vi "ValueChangeTest.vi"() -> ()   [LabVIEW 2016]
uses:
  <vilib>/addons/_JKI Toolkits/Caraya/classes/Assert/Assert Equal Value and Type_Variant.vi
  <vilib>/addons/_JKI Toolkits/Caraya/classes/Assert/Assert.lvclass
  <vilib>/addons/_JKI Toolkits/Caraya/classes/Test/Test.lvclass
panel:
  out "error out":errorcluster
  in  "error in":errorcluster
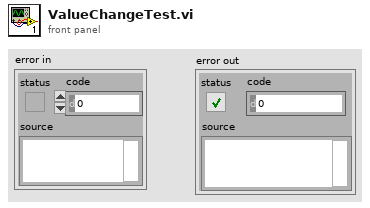
[diagram p1: front panel]
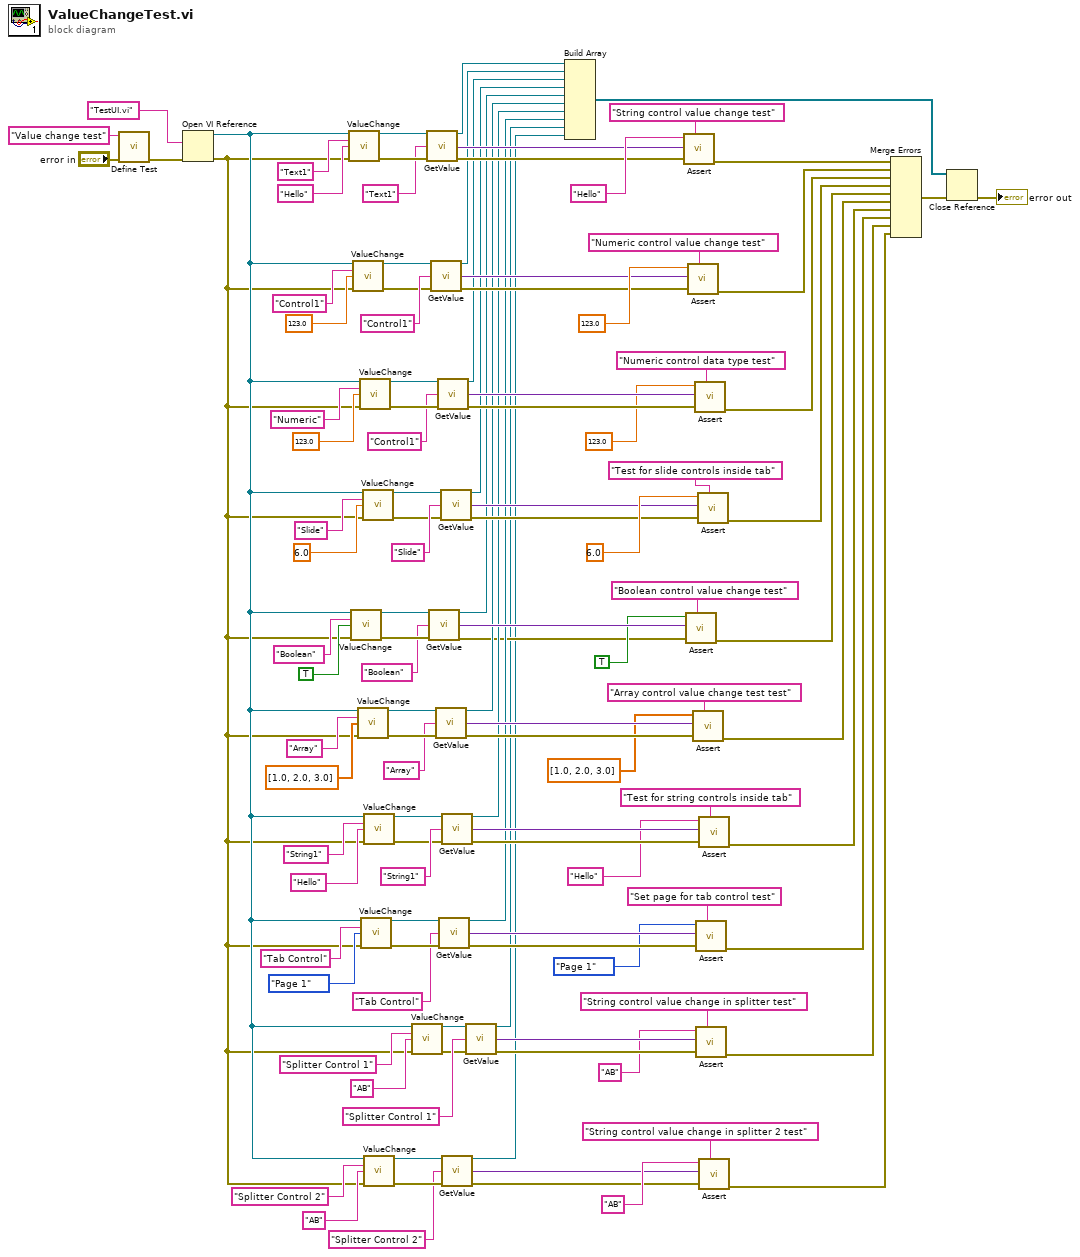
[diagram p0: block diagram]
diagram:
  n1 = call <vilib>:"Define Test.vi"("error in (no error)"="error in", "Label (VI Title)"="Value change test") -> ("error out"=w111:errorcluster)  [unwired: 9 in]
  n2 = Open VI Reference(vi path="TestUI.vi", error in (no error)=w111) -> (vi reference=w4:refnum<vi>, error out=w3:errorcluster)  [unwired: 4 in]
  n3 = call "ValueChange.vi"("VI Reference"=w4, "Control Name"="Text1", "Value"="Hello" ("Control Name"), "error in"=w3) -> ("reference out"=w109:refnum<vi>, "error out"=w118:errorcluster)  [unwired: 10 in]
  n4 = call "ValueChange.vi"("VI Reference"=w4, "Control Name"="Boolean", "Value"=TRUE, "error in"=w3) -> ("reference out"=w73:refnum<vi>, "error out"=w72:errorcluster)  [unwired: 10 in]
  n5 = call "ValueChange.vi"("VI Reference"=w4, "Control Name"="Control1", "Value"=123.0 ("Control Name"), "error in"=w3) -> ("reference out"=w102:refnum<vi>, "error out"=w103:errorcluster)  [unwired: 10 in]
  n6 = call "ValueChange.vi"("VI Reference"=w4, "Control Name"="Array", "Value"=dbl[] [1.0, 2.0, 3.0], "error in"=w3) -> ("reference out"=w63:refnum<vi>, "error out"=w62:errorcluster)  [unwired: 10 in]
  n7 = call "ValueChange.vi"("VI Reference"=w4, "Control Name"="Numeric", "Value"=123.0 ("Control Name"), "error in"=w3) -> ("reference out"=w93:refnum<vi>, "error out"=w92:errorcluster)  [unwired: 10 in]
  n8 = call "ValueChange.vi"("VI Reference"=w4, "Control Name"="Tab Control", "Value"=enum32{"Page 1", "Page 2", "Page 3"}."Page 1" ("Tab Control"), "error in"=w3) -> ("reference out"=w33:refnum<vi>, "error out"=w32:errorcluster)  [unwired: 10 in]
  n9 = call "ValueChange.vi"("VI Reference"=w4, "Control Name"="Slide", "Value"=6.0 ("Control Name"), "error in"=w3) -> ("reference out"=w80:refnum<vi>, "error out"=w81:errorcluster)  [unwired: 10 in]
  n10 = call "ValueChange.vi"("VI Reference"=w4, "Control Name"="String1", "Value"="Hello" ("Control Name"), "error in"=w3) -> ("reference out"=w53:refnum<vi>, "error out"=w54:errorcluster)  [unwired: 10 in]
  n11 = call "ValueChange.vi"("VI Reference"=w4, "Control Name"="Splitter Control 2", "Value"="AB", "error in"=w3) -> ("reference out"=w9:refnum<vi>, "error out"=w8:errorcluster)  [unwired: 10 in]
  n12 = call "ValueChange.vi"("VI Reference"=w4, "Control Name"="Splitter Control 1", "Value"="AB", "error in"=w3) -> ("reference out"=w21:refnum<vi>, "error out"=w22:errorcluster)  [unwired: 10 in]
  n13 = call "GetValue.vi"("VI Reference"=w109, "Control Name"="Text1", "error in"=w118) -> ("VI Reference out"=w44:refnum<vi>, "Control Value"=w100:variant, "error out"=w101:errorcluster)  [unwired: 10 in]
  n14 = call "GetValue.vi"("VI Reference"=w73, "Control Name"="Boolean", "error in"=w72) -> ("VI Reference out"=w39:refnum<vi>, "Control Value"=w74:variant, "error out"=w28:errorcluster)  [unwired: 10 in]
  n15 = call "GetValue.vi"("VI Reference"=w102, "Control Name"="Control1", "error in"=w103) -> ("VI Reference out"=w42:refnum<vi>, "Control Value"=w98:variant, "error out"=w99:errorcluster)  [unwired: 10 in]
  n16 = call "GetValue.vi"("VI Reference"=w63, "Control Name"="Array", "error in"=w62) -> ("VI Reference out"=w38:refnum<vi>, "Control Value"=w65:variant, "error out"=w64:errorcluster)  [unwired: 10 in]
  n17 = call "GetValue.vi"("VI Reference"=w93, "Control Name"="Control1", "error in"=w92) -> ("VI Reference out"=w41:refnum<vi>, "Control Value"=w95:variant, "error out"=w94:errorcluster)  [unwired: 10 in]
  n18 = call "GetValue.vi"("VI Reference"=w33, "Control Name"="Tab Control", "error in"=w32) -> ("VI Reference out"=w29:refnum<vi>, "Control Value"=w35:variant, "error out"=w34:errorcluster)  [unwired: 10 in]
  n19 = call "GetValue.vi"("VI Reference"=w80, "Control Name"="Slide", "error in"=w81) -> ("VI Reference out"=w40:refnum<vi>, "Control Value"=w78:variant, "error out"=w79:errorcluster)  [unwired: 10 in]
  n20 = call "GetValue.vi"("VI Reference"=w53, "Control Name"="String1", "error in"=w54) -> ("VI Reference out"=w37:refnum<vi>, "Control Value"=w51:variant, "error out"=w52:errorcluster)  [unwired: 10 in]
  n21 = call "GetValue.vi"("VI Reference"=w9, "Control Name"="Splitter Control 2", "error in"=w8) -> ("VI Reference out"=w2:refnum<vi>, "Control Value"=w11:variant, "error out"=w10:errorcluster)  [unwired: 10 in]
  n22 = call "GetValue.vi"("VI Reference"=w21, "Control Name"="Splitter Control 1", "error in"=w22) -> ("VI Reference out"=w15:refnum<vi>, "Control Value"=w19:variant, "error out"=w20:errorcluster)  [unwired: 10 in]
  n23 = Build Array(w44, w42, w41, w40, w39, w38, w37, w29, w15, w2) -> (w43:refnum<vi>[])
  n24 = call-poly <vilib>:"Assert.vi"("Label"="String control value change test", "error in (no error)"=w101, "Y"=w100, "X"="Hello" ("Control Name")) -> ("error out"=w97:errorcluster)  [unwired: 7 in]
  n25 = call-poly <vilib>:"Assert.vi"("Label"="Boolean control value change test", "error in (no error)"=w28, "Y"=w74, "X"=TRUE) -> ("error out"=w68:errorcluster)  [unwired: 7 in]
  n26 = call-poly <vilib>:"Assert.vi"("Label"="Numeric control value change test", "error in (no error)"=w99, "Y"=w98, "X"=123.0 ("Control Name")) -> ("error out"=w96:errorcluster)  [unwired: 7 in]
  n27 = call-poly <vilib>:"Assert.vi"("Label"="Array control value change test test", "error in (no error)"=w64, "Y"=w65, "X"=dbl[] [1.0, 2.0, 3.0]) -> ("error out"=w57:errorcluster)  [unwired: 7 in]
  n28 = call-poly <vilib>:"Assert.vi"("Label"="Numeric control data type test", "error in (no error)"=w94, "Y"=w95, "X"=123.0 ("Control Name")) -> ("error out"=w86:errorcluster)  [unwired: 7 in]
  n29 = call-poly <vilib>:"Assert.vi"("Label"="Set page for tab control test", "error in (no error)"=w34, "Y"=w35, "X"=enum32{"Page 1", "Page 2", "Page 3"}."Page 1" ("Tab Control")) -> ("error out"=w27:errorcluster)  [unwired: 7 in]
  n30 = call-poly <vilib>:"Assert.vi"("Label"="String control value change in splitter test", "error in (no error)"=w20, "Y"=w19, "X"="AB") -> ("error out"=w14:errorcluster)  [unwired: 7 in]
  n31 = call-poly <vilib>:"Assert.vi"("Label"="Test for slide controls inside tab", "error in (no error)"=w79, "Y"=w78, "X"=6.0 ("Control Name")) -> ("error out"=w76:errorcluster)  [unwired: 7 in]
  n32 = call-poly <vilib>:"Assert.vi"("Label"="Test for string controls inside tab", "error in (no error)"=w52, "Y"=w51, "X"="Hello" ("Label")) -> ("error out"=w47:errorcluster)  [unwired: 7 in]
  n33 = call-poly <vilib>:"Assert.vi"("Label"="String control value change in splitter 2 test", "error in (no error)"=w10, "Y"=w11, "X"="AB") -> ("error out"=w1:errorcluster)  [unwired: 7 in]
  n34 = Merge Errors(w97, w96, w86, w76, w68, w57, w47, w27, w14, w1) -> (w46:errorcluster)
  n35 = Close Reference(reference=w43, error in (no error)=w46) -> (error out=→"error out":errorcluster)
